vi "getData.vi"(7 "LWRS":refnum<class "Web Request.lvclass">, 11 "Last":dbl format="%#_13g") -> ()   [LabVIEW 2014]
uses:
  <vilib>/wsapi/Web Request.lvclass
  Controller/Controls/Notifier Enum.ctl
  reusable/Data/Data.lvclass
  reusable/Data/Read measTime.vi
  Controller/Controller.lvclass
panel:
  out "Array":errorcluster[](array[cluster])
  out "String":string
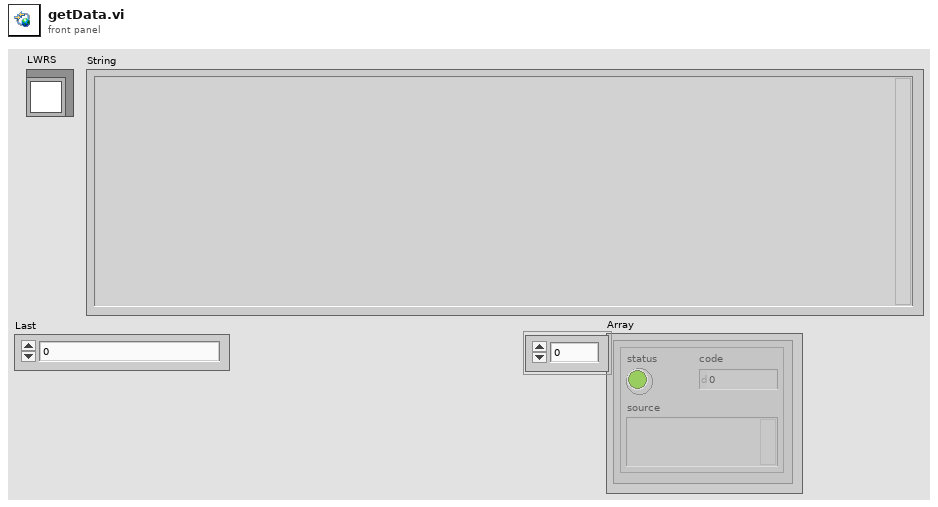
[diagram p1: front panel]
types:
  T1 = typedef "Controller.lvlib/Controller.lvclass/Notifier Enum.ctl" = enum16{"Initialize", "Get", "Set", "Close"}
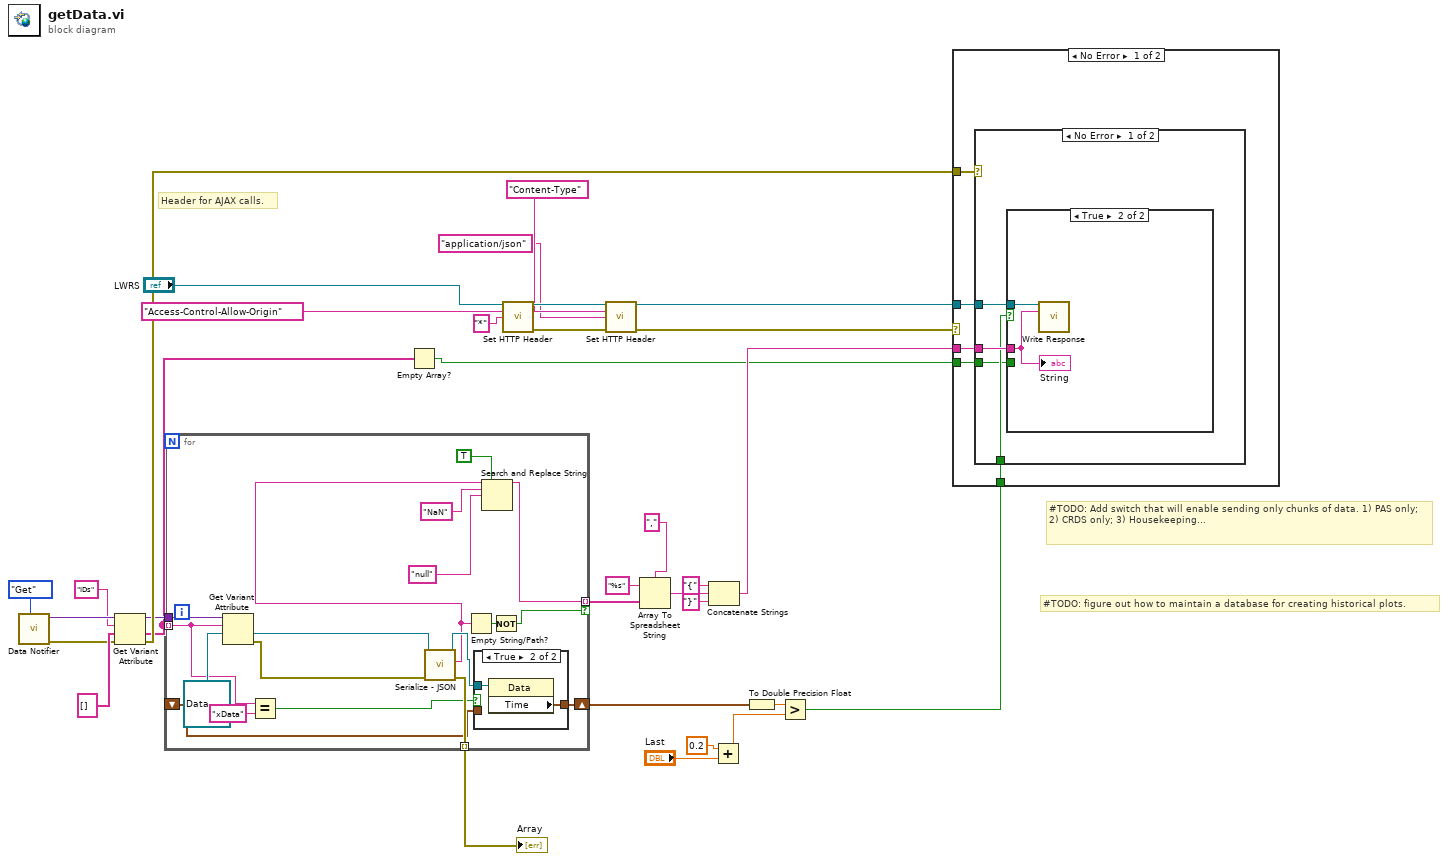
[diagram p0: block diagram]
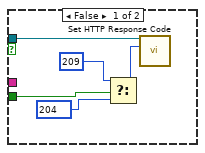
[diagram p3: hidden frame]
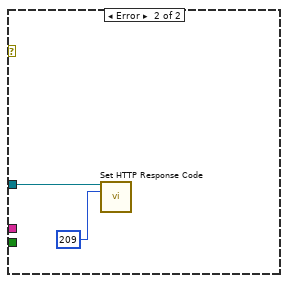
[diagram p4: hidden frame]
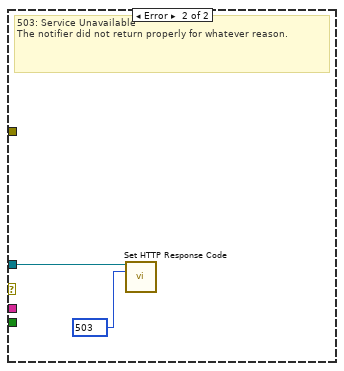
[diagram p5: hidden frame]
diagram:
  # "#TODO: figure out how to maintain a database for creating historical plots."
  # "#TODO: Add switch that will enable sending only chunks of data. 1) PAS only; 2) CRDS only; 3) Housekeeping..."
  # "Header for AJAX calls."
  n1 = call "Data Notifier.vi"("State"=Notifier_Enum."Get") -> ("error out"=w11:errorcluster, "Data Map"=w21:variant)  [unwired: 9 in]
  n2 = Get Variant Attribute(Variant=w21, name="IDs", default value (empty Variant)=string[] [], error in=w11) -> (duplicate Variant=w18:variant, value=w8:string[], error out=w23:errorcluster)  [unwired: 1 out]
  n3 = for {
    tunnel: w8 -> [w34] mode=indexing
    tunnel: w18 -> [w50]
    tunnel: [w41] -> w17 mode=indexing if=w47
    tunnel: [w45] -> w10 mode=indexing
    shift-right: [w37] -> w6
    shift-left: _ -> [w36]
    n4 = Get Variant Attribute(Variant=w50, name=w34, default value (empty Variant)=refnum<class "Data.lvclass"> refnum ("Base Data Lib:Data")) -> (value=w33:refnum<class "Data.lvclass">, error out=w46:errorcluster)  [unwired: 1 in, 2 out]
    n5 = Equal?(x=w34, y="xData") -> (x = y?=w39:bool)
    n6 = call-dynamic "Serialize - JSON.vi"("error in"=w46, "Data in"=w33) -> ("error out"=w45:errorcluster, "Serialized JSON"=w35:string, "Data out"=w38:refnum<class "Data.lvclass">)  [unwired: 7 in]
    n7 = Empty String/Path?(string/path=w35) -> (empty?=w48:bool)
    n8 = case shown="True" w39 {
      tunnel: w38 -> [_ w53]
      tunnel: [w51 w52] -> w37
      tunnel: w36 -> [w51 _]
      frame False {
      }
      frame True {
        n9 = property class="Data"(reference=w53) -> ("Time"=w52:timestamp)  [unwired: 1 in, 2 out]
      }
    }
    n10 = Search and Replace String(replace all?=TRUE ("replace all? (F)"), input string=w35, search string="NaN", replace string="null" ("replace string (\"\")")) -> (result string=w41:string)  [unwired: 4 in, 3 out]
    n11 = Not(x=w48) -> (.not. x?=w47:bool)
  }
  "Array" <- w10
  n12 = Empty Array?(array=w8) -> (empty?=w7:bool)
  n13 = call <vilib>:"Set HTTP Header.vi"("LabVIEW Web Service Request"="LWRS", "header"="Access-Control-Allow-Origin", "header value"="*") -> ("LabVIEW Web Service Request out"=w30:refnum<class "Web Request.lvclass">, "error out"=w29:errorcluster)  [unwired: 11 in]
  n14 = call <vilib>:"Set HTTP Header.vi"("LabVIEW Web Service Request"=w30, "header"="Content-Type", "header value"="application/json", "error in (no error)"=w29) -> ("LabVIEW Web Service Request out"=w25:refnum<class "Web Request.lvclass">, "error out"=w28:errorcluster)  [unwired: 10 in]
  n15 = Array To Spreadsheet String(delimiter (Tab)=",", array=w17, 3:"%s" ("format string")) -> (spreadsheet string=w14:string)
  n16 = Concatenate Strings("{" ("string"), w14, "}" ("string")) -> (w9:string)
  n17 = Add(x=0.2, y="Last") -> (x+y=w3:dbl)
  n18 = To Double Precision Float(number=w6) -> (double precision float=w1:dbl)
  n19 = Greater?(x=w1, y=w3) -> (0:w5:bool)
  n20 = case shown="No Error" w28 {
    tunnel: w23 -> [w58 _]
    tunnel: w25 -> [w57 w73]
    tunnel: w9 -> [w56 _]
    tunnel: w5 -> [w55 _]
    tunnel: w7 -> [w54 _]
    frame No Error {
      n21 = case shown="No Error" w58 {
        tunnel: w57 -> [w62 w71]
        tunnel: w56 -> [w61 _]
        tunnel: w55 -> [w60 _]
        tunnel: w54 -> [w59 _]
        frame No Error {
          # "200: OK"
          n22 = case shown="True" w60 {
            tunnel: w62 -> [w67 w69]
            tunnel: w61 -> [_ w68]
            tunnel: w59 -> [w66 _]
            frame False {
              w65 = 204 items=["100"=100, "101"=101, "200"=200, "201"=201, "202"=202, "203"=203, "204"=204, "205"=205, "206"=206, "300"=300, "301"=301, "302"=302, "303"=303, "304"=304, "305"=305, "306"=306, "307"=307, "400"=400, "401"=401, "402"=402, "403"=403, "404"=404, "405"=405, "406"=406, "407"=407, "408"=408, "409"=409, "410"=410, "411"=411, "412"=412, "413"=413, "414"=414, "415"=415, "416"=416, "417"=417, "500"=500, "501"=501, "502"=502, "503"=503, "504"=504, "505"=505] ("response code (200)")
              n23 = Select(t=209, s=w66, f=w65) -> (s? t:f=w63:i32)
              n24 = call <vilib>:"Set HTTP Response Code.vi"("LabVIEW Web Service Request"=w67, "response code (200)"=w63) -> ()  [unwired: 12 in, 2 out]
            }
            frame True {
              n25 = call <vilib>:"Write Response.vi"("LabVIEW Web Service Request"=w69, "response string"=w68) -> ()  [unwired: 12 in, 2 out]
              "String" <- w68
            }
          }
        }
        frame Error {
          # "204: No Content\nService is valid, DVR is broken"
          n26 = call <vilib>:"Set HTTP Response Code.vi"("LabVIEW Web Service Request"=w71, "response code (200)"=209) -> ()  [unwired: 12 in, 2 out]
        }
      }
    }
    frame Error {
      w72 = 503 items=["100"=100, "101"=101, "200"=200, "201"=201, "202"=202, "203"=203, "204"=204, "205"=205, "206"=206, "300"=300, "301"=301, "302"=302, "303"=303, "304"=304, "305"=305, "306"=306, "307"=307, "400"=400, "401"=401, "402"=402, "403"=403, "404"=404, "405"=405, "406"=406, "407"=407, "408"=408, "409"=409, "410"=410, "411"=411, "412"=412, "413"=413, "414"=414, "415"=415, "416"=416, "417"=417, "500"=500, "501"=501, "502"=502, "503"=503, "504"=504, "505"=505] ("response code (200)")
      # "503: Service Unavailable\nThe notifier did not return properly for whatever reason."
      n27 = call <vilib>:"Set HTTP Response Code.vi"("LabVIEW Web Service Request"=w73, "response code (200)"=w72) -> ()  [unwired: 12 in, 2 out]
    }
  }
